vi "Old Data Replay Run Test.vi"() -> ()   [LabVIEW 2013]
uses:
  Data File Loader/AngleReference.ctl
  <vilib>/rvi/interface/common/niFpgaWaitOnOcc.vi
  <vilib>/rvi/Analysis/host/Private/Sample Rate To Loop Time (ticks).vi
  <vilib>/FPGAPlugInAG/USB-7856R/niLvFpga_Open_USB-7856R.vi
  <vilib>/rvi/interface/common/dynamic/niFpgaDynamicAddResources.vi
  <vilib>/Utility/error.llb/Error Cluster From Error Code.vi
  <vilib>/rvi/errors/niLvFpgaAdjustHostInterfaceError.vi
  <vilib>/FPGAPlugInAG/Dynamic/niLvFpga_Run_Dynamic.vi
  <vilib>/FPGAPlugInAG/Dynamic/niLvFpga_Close_Dynamic.vi
  <vilib>/rvi/interface/nirviOpenFPGA/nirviOpenFPGA.xnode
  FPGA Bitfiles/IPPrototyping_FPGATarget_oldAPU+1oldDataR_qlka9Y0-Q-I.lvbitx
  Compile Tests/old APU + 1 old Data Replay.vi
  <vilib>/rvi/interface/nirviReadWriteControl/nirviReadWriteControl.xnode
  <vilib>/rvi/interface/nirviMethod/nirviMethod.xnode
  <vilib>/rvi/interface/nirviCloseFPGA/nirviCloseFPGA.xnode
  <userlib>/AES/RT/AES RT.lvlib
  <vilib>/rvi/Analysis/host/Public/NI_FpgaMspHost.lvlib
  NiFpgaLv.dll
  <vilib>/rvi/interface/Simulation/niFpgaSimulationCallBeginRW.vi
panel:
  out "Load time (s)":dbl
  in  "RPM Threshold":dbl format="%#_15g"
  in  "Offset":dbl format="%#_15g"
  in  "Reverse Negate":bool
  in  "RPM":dbl format="%#_15g"
  in  "stop":bool
  in  "threshold speed (RPM)":dbl
  in  "threshold voltage":dbl
  in  "maximum speed (RPM)":dbl=10000.0
  in  "maximum voltage":dbl=10.0
  in  "acceleration (RPM/sec)":dbl=inf
  out "Data":dbl[](graph)
  in  "votlage at max RPM":dbl=10.0
  out "Selected Offset":i32
  out "Selected Length":i32
  in  "CycleAngle?":T1
  in  "ReverseData":bool
  in  "MissingTeeth Location":dbl=200.0
  in  "File Path":path=path "C:/Users/sbarrett/Documents/SVN/Engine Simulation/Engine Sim FPGA Example/crank VR data.csv"
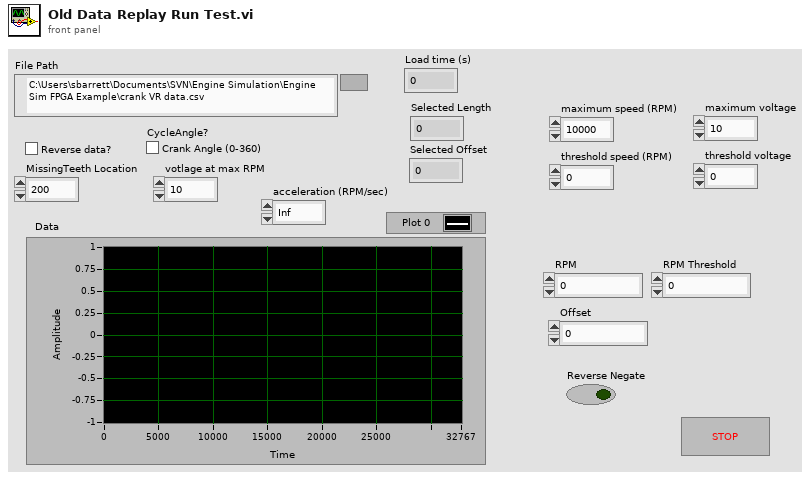
[diagram p1: front panel]
types:
  T1 = typedef "AngleReference.ctl" = bool
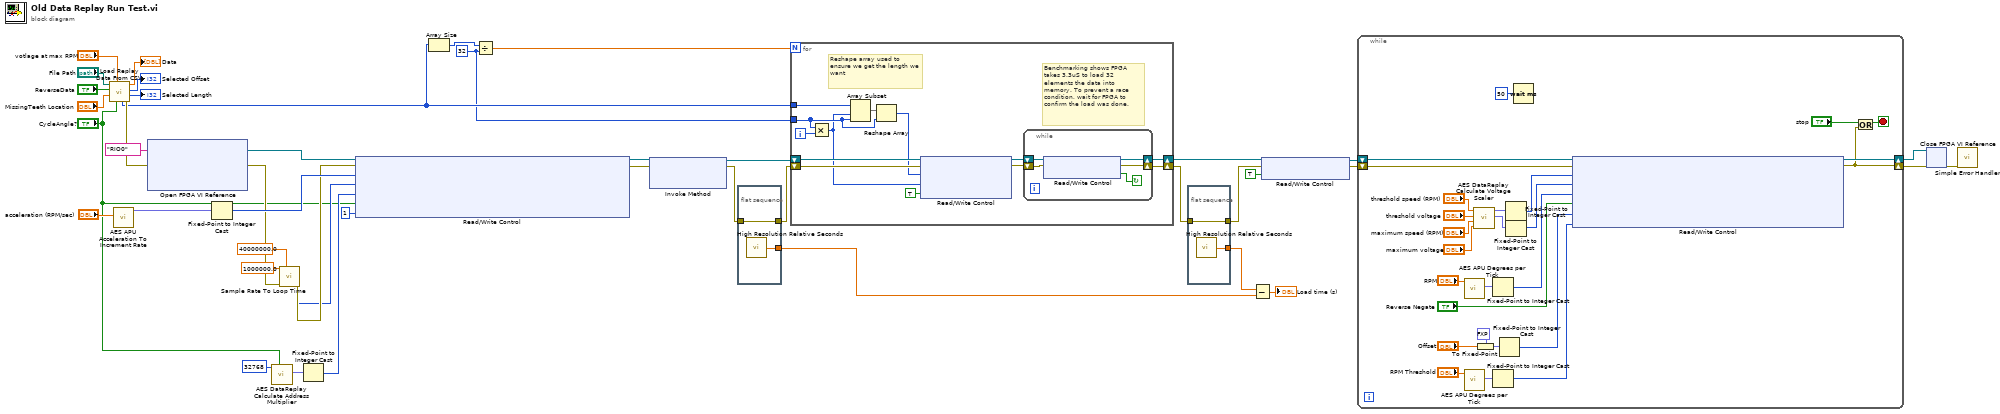
[diagram p0: block diagram]
diagram:
  w1 = 32 ("y")
  n1 = call "Load Replay Data From CSV.vi"("CycleAngle?"="CycleAngle?", "votlage at max RPM"="votlage at max RPM", "MissingTeeth Location"="MissingTeeth Location", "ReverseData"="ReverseData", "File Path"="File Path") -> ("error out"=w27:errorcluster, "Selected Length"=→"Selected Length":i32, "Selected Offset"=→"Selected Offset":i32, "Data"=→"Data":dbl[], "DAC data"=w26:i16[])  [unwired: 2 in]
  n2 = call <userlib>:"AES APU Acceleration To Increment Rate.vi"("acceleration (RPM/sec)"="acceleration (RPM/sec)") -> ("increment rate"=w34:fxp<+/-,47,-4>)  [unwired: 10 in]
  n3 = xnode "Open FPGA VI Reference"("error in"=w27, "resource name"=tag "RIO0") -> ("FPGA VI Reference Out"=w36:refnum<k20>, "error out"=w32:errorcluster)
  n4 = Fixed-Point to Integer Cast(1:w34) -> (0:w33:i64)
  n5 = call <userlib>:"AES DataReplay Calculate Address Multiplier.vi"("CycleAngle?"="CycleAngle?", "memory size (divisible by 32)"=32768) -> ("angle to address multiplier"=w20:fxp<+,18,7>)  [unwired: 9 in]
  n6 = call-poly <vilib>:"Sample Rate To Loop Time.vi"("sample rate (S/s)"=1000000.0, "FPGA clock rate (Hz)"=40000000.0, "error in (no error)"=w32) -> ("count (ticks/S)"=w29:u32, "error out"=w31:errorcluster)  [unwired: 10 in, 1 out]
  n7 = Fixed-Point to Integer Cast(1:w20) -> (0:w19:u32)
  n8 = xnode "Read/Write Control"("FPGA VI Reference In"=w36, "error in"=w31, "APU.Increment Rate"=w33, "DataReplay.UpdateRate.<LOOP NAME>"=w29, "DataReplay.AngleToAddress.<LOOP NAME>.<REPLAY NAME>.<NUMBER>"=w19, "DataReplay.CycleAngle?.<LOOP NAME>.<REPLAY NAME>.<NUMBER>"="CycleAngle?", "DataReplay.Select"=i8 1) -> ("FPGA VI Reference Out"=w23:refnum<k20>, "error out"=w28:errorcluster)
  n9 = Array Size(array=w26) -> (size(s)=w24:i32)
  n10 = Divide(x=w24, y=w1) -> (x/y=w25:dbl)
  n11 = xnode "Invoke Method"("FPGA VI Reference In"=w23, "error in"=w28) -> ("FPGA VI Reference Out"=w22:refnum<k20>, "error out"=w12:errorcluster)  [unwired: 1 in]
  n12 = flat-sequence {
    tunnel: [w46] -> w13
    tunnel: w12 -> [w46]
    tunnel: [w45] -> w8
    frame #0 {
      n13 = call <vilib>:"High Resolution Relative Seconds.vi"() -> ("relative seconds"=w45:dbl)
    }
  }
  n14 = for {
    N: w25 -> [_]
    shift-right: [w56] -> w11
    shift-left: w13 -> [w54]
    tunnel: w26 -> [w59]
    tunnel: w1 -> [w55]
    shift-right: [w47] -> w5
    shift-left: w22 -> [w53]
    i -> [w57]
    # "Reshape array used to ensure we get the length we want"
    # "Benchmarking shows FPGA takes 3.3uS to load 32 elements the data into memory. To prevent a race condition, wait for FPGA to confirm the load was done."
    n15 = Multiply(x=w55, y=w57) -> (x*y=w51:i32)
    n16 = Array Subset(array=w59, index=w51, length=w55) -> (w58:i16[])
    n17 = Reshape Array(w58, w55) -> (w52:i16[])
    n18 = xnode "Read/Write Control"("FPGA VI Reference In"=w53, "error in"=w54, "DataReplay.Data"=w52, "DataReplay.LoadOffset"=w51, "DataReplay.Toggle"=TRUE) -> ("FPGA VI Reference Out"=w49:refnum<k20>, "error out"=w48:errorcluster)
    n19 = while {
      shift-right: [w62] -> w56
      shift-left: w48 -> [w64]
      shift-right: [w60] -> w47
      shift-left: w49 -> [w63]
      stop <- w61 continue-if-true
      n20 = xnode "Read/Write Control"("FPGA VI Reference In"=w63, "error in"=w64) -> ("FPGA VI Reference Out"=w60:refnum<k20>, "error out"=w62:errorcluster, "DataReplay.Toggle"=w61:bool)
    }
  }
  n21 = flat-sequence {
    tunnel: [w66] -> w10
    tunnel: w11 -> [w66]
    tunnel: [w65] -> w9
    frame #0 {
      n22 = call <vilib>:"High Resolution Relative Seconds.vi"() -> ("relative seconds"=w65:dbl)
    }
  }
  n23 = Subtract(x=w9, y=w8) -> (x-y=→"Load time (s)":dbl)
  n24 = xnode "Read/Write Control"("FPGA VI Reference In"=w5, "error in"=w10, "DataReplay.LoadDone"=TRUE) -> ("FPGA VI Reference Out"=w4:refnum<k20>, "error out"=w6:errorcluster)
  n25 = while {
    shift-right: [w71] -> w17
    shift-left: w6 -> [w92]
    shift-right: [w82] -> w16
    shift-left: w4 -> [w91]
    stop <- w72 stop-if-true
    n26 = call <userlib>:"AES APU Degrees per Tick.vi"("RPM"="RPM") -> ("degrees per tick"=w79:fxp<+/-,47,-4>)  [unwired: 9 in, 1 out]
    n27 = call <userlib>:"AES APU Degrees per Tick.vi"("RPM"="RPM Threshold") -> ("degrees per tick"=w70:fxp<+/-,47,-4>)  [unwired: 9 in, 1 out]
    n28 = call <userlib>:"AES DataReplay Calculate Voltage Scaler.vi"("maximum voltage"="maximum voltage", "maximum speed (RPM)"="maximum speed (RPM)", "threshold voltage"="threshold voltage", "threshold speed (RPM)"="threshold speed (RPM)") -> ("intercept (b)"=w85:fxp<+/-,18,3>, "slope (m)"=w86:fxp<+,18,12>)  [unwired: 6 in]
    n29 = To Fixed-Point(fixed-point type=fxp<+/-,61,10> 0.0 ("FullyCustomTeeth.Cams.Cam1.Offset"), number="Offset") -> (fixed-point=w75:fxp<+/-,61,10>)
    n30 = Fixed-Point to Integer Cast(1:w79) -> (0:w78:i64)
    n31 = Fixed-Point to Integer Cast(1:w70) -> (0:w68:i64)
    n32 = Fixed-Point to Integer Cast(1:w75) -> (0:w73:i64)
    n33 = Fixed-Point to Integer Cast(1:w86) -> (0:w84:u32)
    n34 = Fixed-Point to Integer Cast(1:w85) -> (0:w83:i32)
    n35 = Wait (ms)(milliseconds to wait=u32 50) -> ()  [unwired: 1 out]
    n36 = xnode "Read/Write Control"("FPGA VI Reference In"=w91, "error in"=w92, "DataReplay.VScaleSlope.<LOOP NAME>.<REPLAY NAME>.<NUMBER>"=w84, "DataReplay.VScaleIntercept.<LOOP NAME>.<REPLAY NAME>.<NUMBER>"=w83, "APU.Degrees per Tick"=w78, "DataReplay.ReverseNegate?.<LOOP NAME>.<REPLAY NAME>.<NUMBER>"="Reverse Negate", "DataReplay.Offset.<LOOP NAME>.<REPLAY NAME>.<NUMBER>"=w73, "DataReplay.RPMThreshold.<LOOP NAME>.<REPLAY NAME>.<NUMBER>"=w68) -> ("FPGA VI Reference Out"=w82:refnum<k20>, "error out"=w71:errorcluster)
    n37 = Or(x="stop", y=w71) -> (x .or. y?=w72:bool)
  }
  n38 = xnode "Close FPGA VI Reference"("FPGA VI Reference In"=w16, "error in"=w17) -> ("error out"=w15:errorcluster)
  n39 = call <vilib>:"Simple Error Handler.vi"("error in (no error)"=w15) -> ()  [unwired: 4 in, 5 out]
